vi "Reinitialise.vi"(8 "error in":errorcluster, 10 "Value":T1, 11 "References in":T2) -> (0 "error out":errorcluster)   [LabVIEW 2019]
uses:
  TypeDef/#TypeDef_References.ctl
  TypeDef/#TypeDef_Buttons.ctl
  TypeDef/#TypeDef_ReferencesMeassurementProp.ctl
  TypeDef/#TypeDef_ReferencesArchiveProp.ctl
  TypeDef/#TypeDef_Lists.ctl
  TypeDef/#TypeDef_MeasProp.ctl
  TypeDef/#TypeDef_OpProp.ctl
  TypeDef/#TypeDef_Enum_ModeOp.ctl
  TypeDef/#TypeDef_Enum_Buttons.ctl
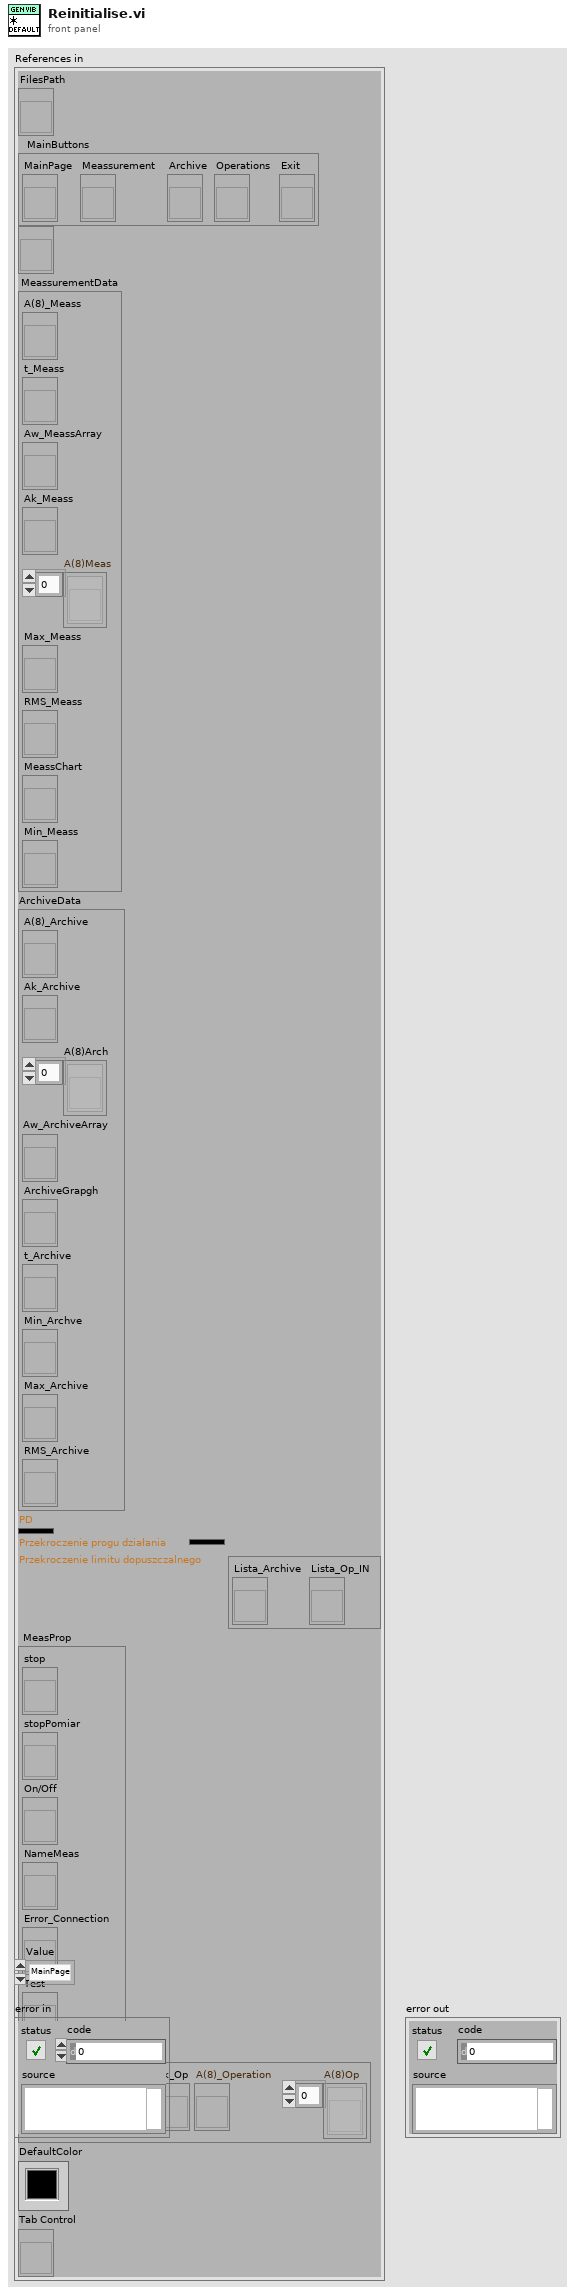
[diagram p1: front panel]
types:
  T1 = typedef "#TypeDef_Enum_Buttons.ctl" = enum32{"MainPage", "Pomiar", "Archiwum", "Operacje", "Wyjœcie"}
  T2 = typedef "#TypeDef_References.ctl" = cluster{"FilesPath":refnum<vi>, "MainButtons":T3, "Lista CTRL":refnum<vi>, "MeassurementData":T4, "ArchiveData":T5, "PD":u32, "LD":u32, "Lists":T6, "MeasProp":T7, "OpProp":T8, "DefaultColor":u32, "Tab Control":refnum<vi>}
  T3 = typedef "#TypeDef_Buttons.ctl" = cluster{"MainPage":refnum<vi>, "Meassurement":refnum<vi>, "Archive":refnum<vi>, "Operations":refnum<vi>, "Exit":refnum<vi>}
  T4 = typedef "#TypeDef_ReferencesMeassurementProp.ctl" = cluster{"A(8)_Meass":refnum<vi>, "t_Meass":refnum<vi>, "Aw_MeassArray":refnum<vi>, "Ak_Meass":refnum<vi>, "A(8)Meas":refnum<vi>[], "Max_Meass":refnum<vi>, "RMS_Meass":refnum<vi>, "MeassChart":refnum<vi>, "Min_Meass":refnum<vi>}
  T5 = typedef "#TypeDef_ReferencesArchiveProp.ctl" = cluster{"A(8)_Archive":refnum<vi>, "Ak_Archive":refnum<vi>, "A(8)Arch":refnum<vi>[], "Aw_ArchiveArray":refnum<vi>, "ArchiveGrapgh":refnum<vi>, "t_Archive":refnum<vi>, "Min_Archve":refnum<vi>, "Max_Archive":refnum<vi>, "RMS_Archive":refnum<vi>}
  T6 = typedef "#TypeDef_Lists.ctl" = cluster{"Lista_Archive":refnum<vi>, "Lista_Op_IN":refnum<vi>}
  T7 = typedef "#TypeDef_MeasProp.ctl" = cluster{"stop":refnum<vi>, "stopPomiar":refnum<vi>, "On/Off":refnum<vi>, "NameMeas":refnum<vi>, "Error_Connection":refnum<vi>, "Test":refnum<vi>}
  T8 = typedef "#TypeDef_OpProp.ctl" = cluster{"Name_Op":refnum<vi>, "t_Op":refnum<vi>, "Modu³":refnum<vi>, "Ak_Op":refnum<vi>, "A(8)_Operation":refnum<vi>, "A(8)Op":refnum<vi>[]}
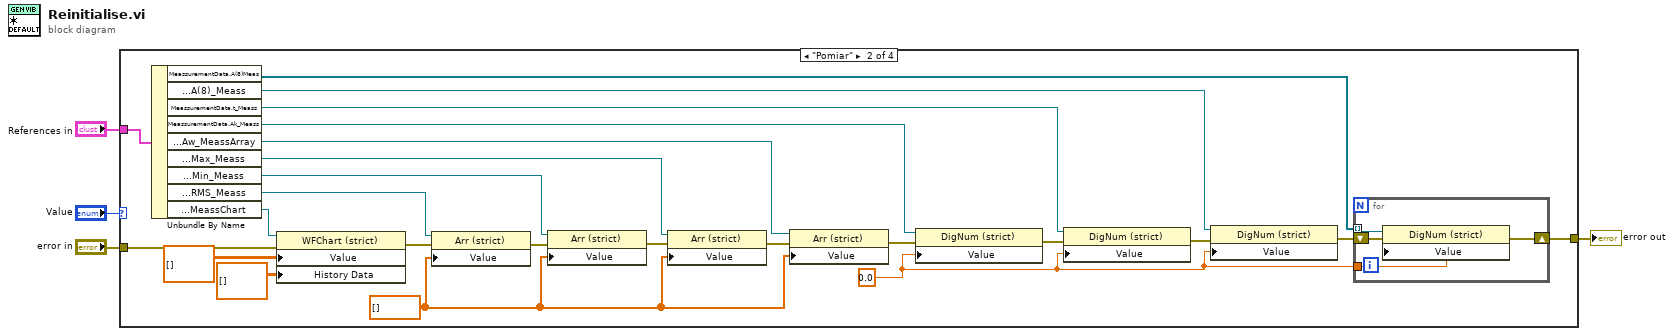
[diagram p0: block diagram]
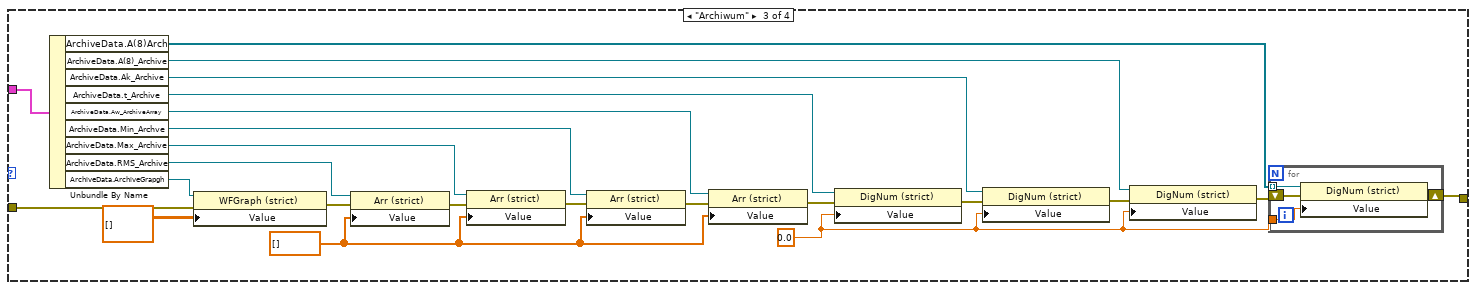
[diagram p3: hidden frame]
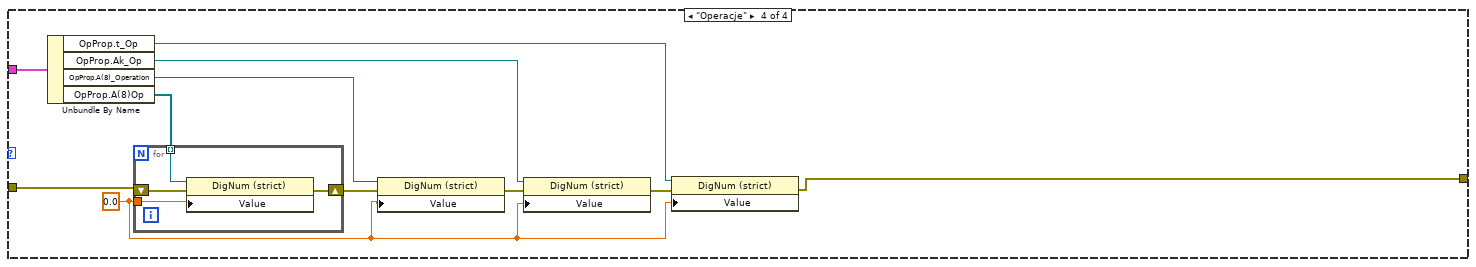
[diagram p4: hidden frame]
diagram:
  n1 = case shown="\"Pomiar\"" "Value" {
    tunnel: "References in" -> [_ w29 w56 w71]
    tunnel: [w5 w8 w35 w61] -> w4
    tunnel: "error in" -> [w5 w11 w46 w69]
    frame "MainPage", Default {
    }
    frame "Pomiar" {
      w7 = 0.0 ("Value")
      w19 = dbl[] [] ("Value")
      n2 = Unbundle By Name(w29) -> ("MeassurementData.A(8)Meas"=w9:refnum<vi>[], "MeassurementData.A(8)_Meass"=w12:refnum<vi>, "MeassurementData.t_Meass"=w14:refnum<vi>, "MeassurementData.Ak_Meass"=w16:refnum<vi>, "MeassurementData.Aw_MeassArray"=w20:refnum<vi>, "MeassurementData.Max_Meass"=w21:refnum<vi>, "MeassurementData.Min_Meass"=w23:refnum<vi>, "MeassurementData.RMS_Meass"=w26:refnum<vi>, "MeassurementData.MeassChart"=w28:refnum<vi>)
      n3 = property class="WFChart (strict)"(reference=w28, error in=w11, "Value"=dbl[][] [], "History Data"=dbl[][] []) -> (error out=w25:errorcluster)  [unwired: 1 out]
      n4 = property class="Arr (strict)"(reference=w26, error in=w25, "Value"=w19) -> (error out=w24:errorcluster)  [unwired: 1 out]
      n5 = property class="Arr (strict)"(reference=w23, error in=w24, "Value"=w19) -> (error out=w22:errorcluster)  [unwired: 1 out]
      n6 = property class="Arr (strict)"(reference=w21, error in=w22, "Value"=w19) -> (error out=w18:errorcluster)  [unwired: 1 out]
      n7 = property class="Arr (strict)"(reference=w20, error in=w18, "Value"=w19) -> (error out=w17:errorcluster)  [unwired: 1 out]
      n8 = property class="DigNum (strict)"(reference=w16, error in=w17, "Value"=w7) -> (error out=w15:errorcluster)  [unwired: 1 out]
      n9 = property class="DigNum (strict)"(reference=w14, error in=w15, "Value"=w7) -> (error out=w13:errorcluster)  [unwired: 1 out]
      n10 = property class="DigNum (strict)"(reference=w12, error in=w13, "Value"=w7) -> (error out=w10:errorcluster)  [unwired: 1 out]
      n11 = for {
        tunnel: w9 -> [w32] mode=indexing
        shift-right: [w31] -> w8
        shift-left: w10 -> [w33]
        tunnel: w7 -> [w30]
        n12 = property class="DigNum (strict)"(reference=w32, error in=w33, "Value"=w30) -> (error out=w31:errorcluster)  [unwired: 1 out]
      }
    }
    frame "Archiwum" {
      w34 = 0.0 ("Value")
      w51 = dbl[] [] ("Value")
      n13 = Unbundle By Name(w56) -> ("ArchiveData.A(8)Arch"=w36:refnum<vi>[], "ArchiveData.A(8)_Archive"=w39:refnum<vi>, "ArchiveData.Ak_Archive"=w40:refnum<vi>, "ArchiveData.t_Archive"=w41:refnum<vi>, "ArchiveData.Aw_ArchiveArray"=w38:refnum<vi>, "ArchiveData.Min_Archve"=w42:refnum<vi>, "ArchiveData.Max_Archive"=w43:refnum<vi>, "ArchiveData.RMS_Archive"=w44:refnum<vi>, "ArchiveData.ArchiveGrapgh"=w45:refnum<vi>)
      n14 = property class="WFGraph (strict)"(reference=w45, error in=w46, "Value"=dbl[][] []) -> (error out=w54:errorcluster)  [unwired: 1 out]
      n15 = property class="Arr (strict)"(reference=w44, error in=w54, "Value"=w51) -> (error out=w53:errorcluster)  [unwired: 1 out]
      n16 = property class="Arr (strict)"(reference=w43, error in=w53, "Value"=w51) -> (error out=w52:errorcluster)  [unwired: 1 out]
      n17 = property class="Arr (strict)"(reference=w42, error in=w52, "Value"=w51) -> (error out=w50:errorcluster)  [unwired: 1 out]
      n18 = property class="Arr (strict)"(reference=w38, error in=w50, "Value"=w51) -> (error out=w49:errorcluster)  [unwired: 1 out]
      n19 = property class="DigNum (strict)"(reference=w41, error in=w49, "Value"=w34) -> (error out=w48:errorcluster)  [unwired: 1 out]
      n20 = property class="DigNum (strict)"(reference=w40, error in=w48, "Value"=w34) -> (error out=w47:errorcluster)  [unwired: 1 out]
      n21 = property class="DigNum (strict)"(reference=w39, error in=w47, "Value"=w34) -> (error out=w37:errorcluster)  [unwired: 1 out]
      n22 = for {
        tunnel: w36 -> [w59] mode=indexing
        shift-right: [w58] -> w35
        shift-left: w37 -> [w60]
        tunnel: w34 -> [w57]
        n23 = property class="DigNum (strict)"(reference=w59, error in=w60, "Value"=w57) -> (error out=w58:errorcluster)  [unwired: 1 out]
      }
    }
    frame "Operacje" {
      w63 = 0.0 ("Value")
      n24 = Unbundle By Name(w71) -> ("OpProp.t_Op"=w62:refnum<vi>, "OpProp.Ak_Op"=w65:refnum<vi>, "OpProp.A(8)_Operation"=w67:refnum<vi>, "OpProp.A(8)Op"=w70:refnum<vi>[])
      n25 = for {
        tunnel: w70 -> [w75] mode=indexing
        shift-right: [w74] -> w68
        shift-left: w69 -> [w73]
        tunnel: w63 -> [w72]
        n26 = property class="DigNum (strict)"(reference=w75, error in=w73, "Value"=w72) -> (error out=w74:errorcluster)  [unwired: 1 out]
      }
      n27 = property class="DigNum (strict)"(reference=w67, error in=w68, "Value"=w63) -> (error out=w66:errorcluster)  [unwired: 1 out]
      n28 = property class="DigNum (strict)"(reference=w65, error in=w66, "Value"=w63) -> (error out=w64:errorcluster)  [unwired: 1 out]
      n29 = property class="DigNum (strict)"(reference=w62, error in=w64, "Value"=w63) -> (error out=w61:errorcluster)  [unwired: 1 out]
    }
  }
  "error out" <- w4
